vi "Get Pane Height.vi"(8 "error in (no error)":errorcluster caption="entrée d'erreur (pas d'erreur)", 11 "UI Cam Basler en entrée":refnum<class "UI Cam Basler.lvclass">) -> (0 "error out":errorcluster caption="sortie d'erreur", 3 "UI Cam Basler en sortie":refnum<class "UI Cam Basler.lvclass">)   [LabVIEW 2023, in "UI Cam Basler.lvclass"]
uses:
  UI Cam Basler.lvclass
  UI Cam Basler.lvclass/UI Cam Basler.ctl
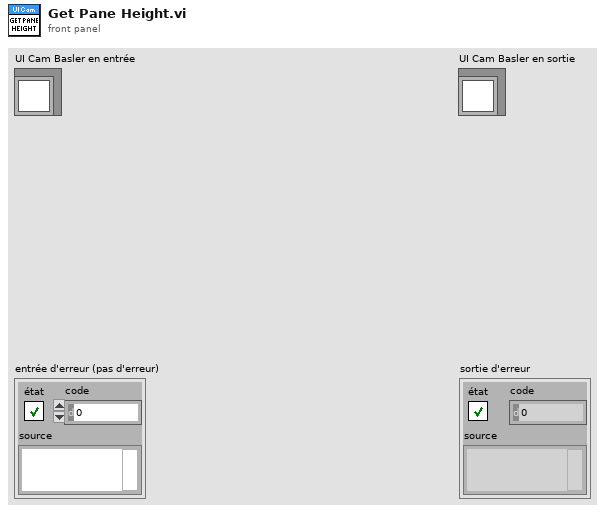
[diagram p1: front panel]
types:
  T1 = typedef "LVBoundsTypeDef.ctl" = cluster{"Width":u32, "Height":u32}
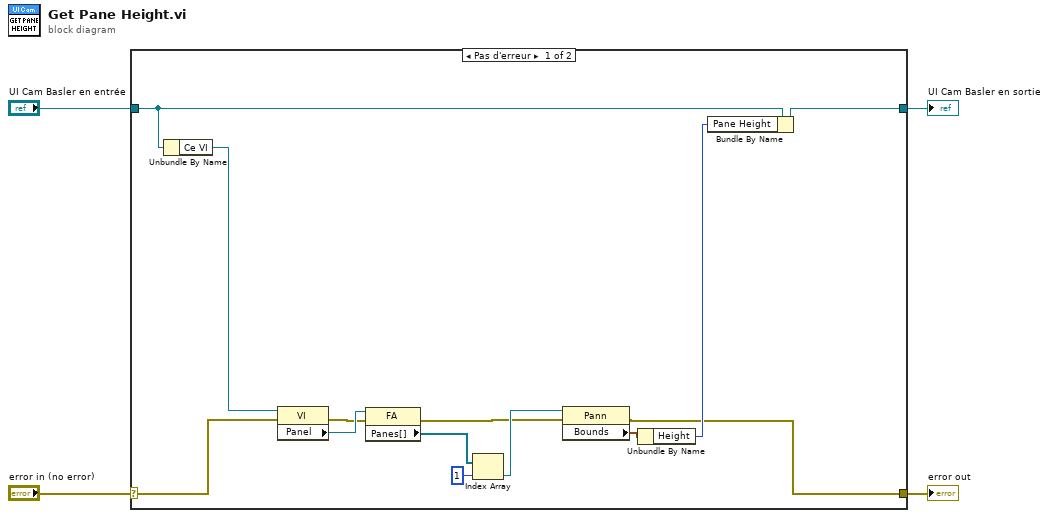
[diagram p0: block diagram]
diagram:
  n1 = case shown="Pas d'erreur" "error in (no error)" {
    selector: "error in (no error)" -> [w9 w19]
    tunnel: [w5 w19] -> w3
    tunnel: [w17 w18] -> w1
    tunnel: "UI Cam Basler en entrée" -> [w16 w18]
    frame No Error {
      n2 = Unbundle By Name(w16) -> ("Ce VI"=w10:refnum<vi>)
      n3 = property class="VI"(reference=w10, error in=w9) -> (error out=w7:errorcluster, "Panel"=w15:refnum<vi>)  [unwired: 1 out]
      n4 = property class="FA"(reference=w15, error in=w7) -> (error out=w6:errorcluster, "Panes[]"=w14:refnum<vi>[])  [unwired: 1 out]
      n5 = Index Array(array=w14, index=1 ("indice")) -> (element=w12:refnum<vi>)
      n6 = property class="Pann"(reference=w12, error in=w6) -> (error out=w5:errorcluster, "Bounds"=w11:T1)  [unwired: 1 out]
      n7 = Unbundle By Name(w11) -> ("Height"=w8:u32)
      n8 = Bundle By Name(cluster=w16, "Pane Height"=w8) -> (w17:refnum<class "UI Cam Basler.lvclass">)
    }
    frame Error {
    }
  }
  "error out" <- w3
  "UI Cam Basler en sortie" <- w1
